vi "tester_calc_conveyor_single_module.vi"() -> ()   [LabVIEW 2011]
uses:
  Conveyor module state.ctl
panel:
  in  "Next Iteration":bool
  out "Lifter Module State":T1
  out "Conveyor Speed":dbl
  out "Accepting Balls":bool
  in  "Ball is out":bool
  in  "Push Ball Out":bool
  in  "Load Speed":dbl=1.0
  in  "Adjust Speed":dbl=0.2
  in  "Ball Detector Count":i32
  in  "Reset":bool
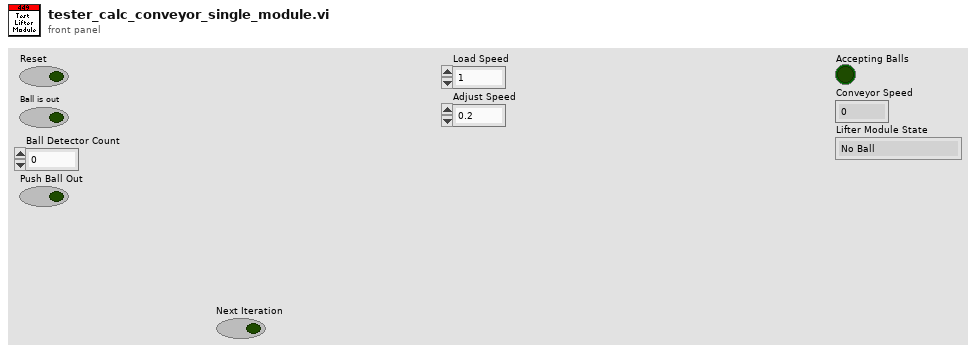
[diagram p1: front panel]
types:
  T1 = typedef "Conveyor module state.ctl" = enum16{"No Ball", "Has Ball", "Ball Below Hold", "Ball Above Hold", "Outputting Ball", "Reset"}
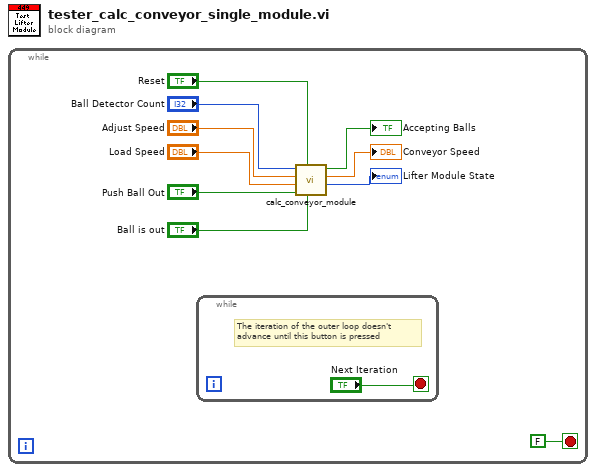
[diagram p0: block diagram]
diagram:
  n1 = while {
    stop <- FALSE stop-if-true
    n2 = while {
      stop <- "Next Iteration" stop-if-true
      # "The iteration of the outer loop doesn't\nadvance until this button is pressed"
    }
    n3 = call "calc_conveyor_module.vi"("Ball is out"="Ball is out", "Reset"="Reset", "Push Ball Out"="Push Ball Out", "Load Speed"="Load Speed", "Adjust Speed"="Adjust Speed", "Ball Detector Count"="Ball Detector Count") -> ("Lifter Module State"=→"Lifter Module State":T1, "Conveyor Speed"=→"Conveyor Speed":dbl, "Accepting Balls"=→"Accepting Balls":bool)  [unwired: 3 in]
  }
